vi "Configure Measurement Correction.vi"(0 "VISA resource name":refnum<visa-resource-name>, 1 "correction method short)":u16(ring) items=["short", "open", "load"], 5 "enable correction (T)":bool=TRUE, 11 "error in (no error)":errorcluster, 12 "reference value I (1.000E+4)":dbl=10000.0 min=-1000000000.0 max=1000000000.0 step=1.0 format="%.3e", 13 "reference value II (1.000E+4)":dbl=10000.0 min=-1000000000.0 max=1000000000.0 step=1.0 format="%.3e") -> (4 "VISA resource name out":refnum<visa-resource-name>, 15 "error out":errorcluster)   [LabVIEW 2016, in "Agilent 4263X.lvlib"]
doc: "This VI configures the correction mode of the instrument."
uses:
  <instrlib>/Agilent 4263X/Agilent 4263X.lvlib
panel:
  # "on \noff"
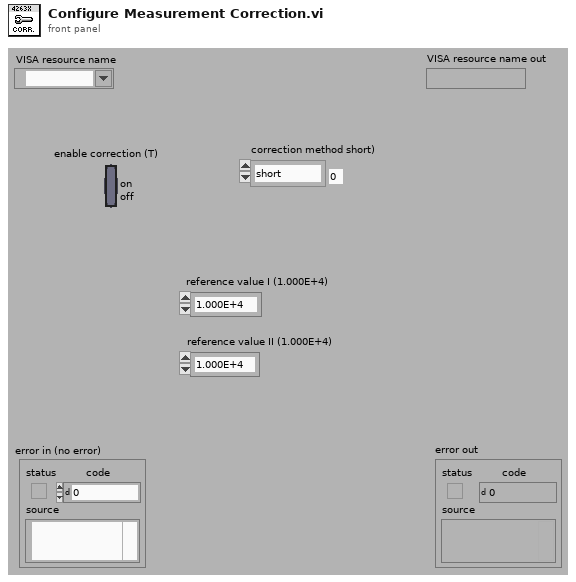
[diagram p1: front panel]
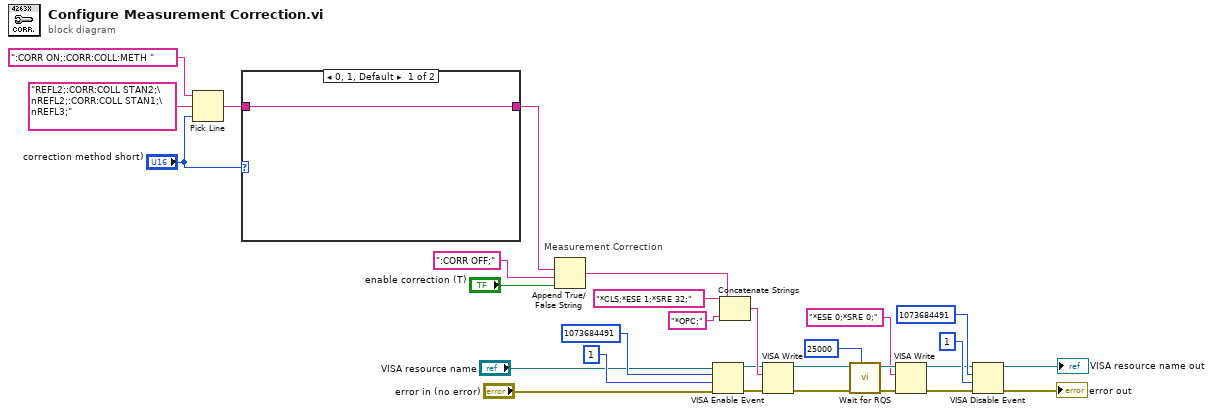
[diagram p0: block diagram]
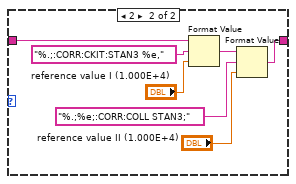
[diagram p2: hidden frame]
diagram:
  # "Measurement Correction"
  n1 = Pick Line(string ("")=":CORR ON;:CORR:COLL:METH ", multi-line string="REFL2;:CORR:COLL STAN2;\nREFL2;:CORR:COLL STAN1;\nREFL3;", line index="correction method short)") -> (output string=w6:string)
  n2 = case shown="0, 1, Default" "correction method short)" {
    tunnel: w6 -> [w30 w37]
    tunnel: [w30 w31] -> w3
    frame 0, 1, Default {
    }
    frame 2 {
      n3 = Format Value(string ("")=w37, format string="%.;:CORR:CKIT:STAN3 %e,", value (0)="reference value I (1.000E+4)") -> (output string=w34:string)
      n4 = Format Value(string ("")=w34, format string="%.;%e;:CORR:COLL STAN3;", value (0)="reference value II (1.000E+4)") -> (output string=w31:string)
    }
  }
  n5 = Append True/False String(1:"enable correction (T)", 2:":CORR OFF;", 3:w3) -> (0:w2:string)  [unwired: 1 in]
  n6 = VISA Enable Event(8:"error in (no error)", 9:u16 1, 10:u32 1073684491, 11:"VISA resource name") -> (0:w16:errorcluster, 3:w15:refnum<visa-resource-name>)
  n7 = Concatenate Strings("*CLS;*ESE 1;*SRE 32;", w2, "*OPC;") -> (w27:string)
  n8 = VISA Write(VISA resource name=w15, write buffer=w27, error in (no error)=w16) -> (VISA resource name out=w26:refnum<visa-resource-name>, error out=w25:errorcluster)  [unwired: 1 out]
  n9 = call <vilib>:"Wait for RQS.VI"("timeout (25000 ms)"=u32 25000, "error in (no error)"=w25, "VISA resource name"=w26) -> ("error out"=w23:errorcluster, "VISA resource name out"=w24:refnum<visa-resource-name>)  [unwired: 6 in, 1 out]
  n10 = VISA Write(VISA resource name=w24, write buffer="*ESE 0;*SRE 0;", error in (no error)=w23) -> (VISA resource name out=w11:refnum<visa-resource-name>, error out=w12:errorcluster)  [unwired: 1 out]
  n11 = VISA Disable Event(8:w12, 9:u16 1, 10:u32 1073684491, 11:w11) -> (0:→"error out":errorcluster, 3:→"VISA resource name out":refnum<visa-resource-name>)
